vi "ComputeWfmScalar.vi"(6 "GrpCfg":T1, 7 "Speed":T2, 8 "error in (no error)":errorcluster, 10 "Y Array":sgl[](array[numeric]), 11 "Frequency in":refnum<class "Frequency.lvclass">) -> (0 "error out":errorcluster, 2 "Metric":dbl, 3 "Frequency Out":refnum<class "Frequency.lvclass">)   [LabVIEW 2018, in "Measurement Channels.lvlib" / "Frequency.lvclass"]
uses:
  Frequency.lvclass
  C:/Users/Jeff Tipps/Documents/DAQMan/source/Classes/Measurements/Class Channel/Channel.lvclass
  Common/Controls/TE_Designator.ctl
  Common/Controls/Group Timing Info.ctl
  Frequency.lvclass/Frequency.ctl
  Class Channel/Read Scale.vi
  Class Channel/Read Offset.vi
  Class Tachometer/Tachometer.lvclass
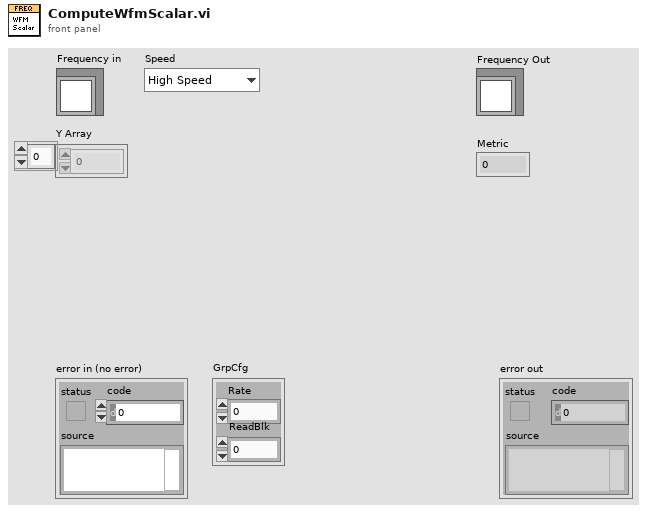
[diagram p1: front panel]
types:
  T1 = typedef "Group Timing Info.ctl" = cluster{"Rate":dbl, "ReadBlk":i32}
  T2 = typedef "TE_Designator.ctl" = enum16{"High Speed", "Low Speed"}
  T3 = cluster{"Analog Tach State":dbl, "Edge Detection State":cluster{"processed data":dbl, "buffer data":dbl[]}, "Reset?":bool}
  T4 = cluster{"state":enum16{"0 Pulses", "1 Pulse", "2+ Pulses"}, "last pulse position":dbl, "RPM":dbl, "Empty Blocks":i32}
  T5 = typedef "OAT Position Info.ctl" = cluster{"positions [s]":dbl[], "samples/rev":dbl}
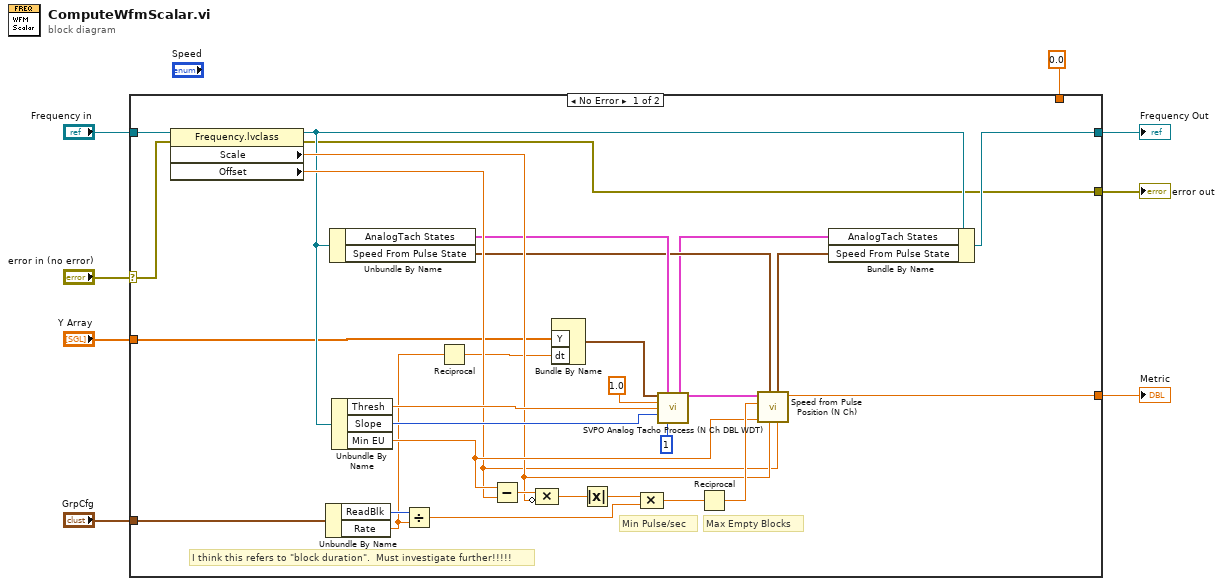
[diagram p0: block diagram]
diagram:
  n1 = case shown="No Error" "error in (no error)" {
    selector: "error in (no error)" -> [w26 w41]
    tunnel: [w28 w40] -> w8
    tunnel: "GrpCfg" -> [w14 _]
    tunnel: "Y Array" -> [w16 _]
    tunnel: "Frequency in" -> [w27 w39]
    tunnel: [w17 w41] -> w3
    tunnel: 0.0 ("Speed in EU") -> [_ w40]
    tunnel: [w18 w39] -> w1
    frame No Error {
      # "I think this refers to \"block duration\".  Must investigate further!!!!!"
      # "Max Empty Blocks"
      # "Min Pulse/sec"
      n2 = property class="Frequency.lvclass"(reference=w27, error in=w26) -> (reference out=w21:refnum<class "Frequency.lvclass">, error out=w17:errorcluster, "Scale"=w25:dbl, "Offset"=w24:dbl)
      n3 = Unbundle By Name(w14) -> ("ReadBlk"=w13:i32, "Rate"=w11:dbl)
      n4 = Unbundle By Name(w21) -> ("AnalogTach States"=w23:T3, "Speed From Pulse State"=w22:T4)
      n5 = Unbundle By Name(w21) -> ("Thresh"=w37:dbl, "Slope"=w36:u16, "Min EU"=w32:dbl)
      n6 = Divide(x=w13, y=w11) -> (x/y=w12:dbl)
      n7 = Reciprocal(x=w11) -> (1/x=w10:dbl)
      n8 = Subtract(x=w32, y=w24) -> (x-y=w29:dbl)
      n9 = Compound Arithmetic op=MULTIPLY(w29, invert w25) -> (w31:dbl)
      n10 = Bundle By Name("Y"=w16, "dt"=w10) -> (w15:waveform(sgl))  [unwired: 1 in]
      n11 = Absolute Value(x=w31) -> (abs(x)=w30:dbl)
      n12 = Compound Arithmetic op=MULTIPLY(w30, w12) -> (w34:dbl)
      n13 = call "SVPO Analog Tacho Process (N Ch DBL WDT).vi"("analog tacho signal"=w15, "AnalogTach States"=w23, "PPR"=1.0, "Thresh(V)"=w37, "Slope"=w36, "pulse width (2)"=1) -> ("AnalogTach States Out"=w20:T3, "speed position info"=w38:T5)  [unwired: 8 in]
      n14 = Reciprocal(x=w34) -> (1/x=w33:dbl)
      n15 = call "Speed from Pulse Position (N Ch).vi"("Offset"=w24, "Scale"=w25, "Speed From Pulse"=w22, "Min EU"=w32, "Max Empty Blocks"=w33, "speed position info"=w38) -> ("Speed in EU"=w28:dbl, "Speed From Pulse"=w19:T4)  [unwired: 4 in]
      n16 = Bundle By Name(cluster=w21, "AnalogTach States"=w20, "Speed From Pulse State"=w19) -> (w18:refnum<class "Frequency.lvclass">)
    }
    frame Error {
    }
  }
  "error out" <- w3
  "Metric" <- w8
  "Frequency Out" <- w1
